vi "SbigExposure.vi"(0 "error in (no error)":errorcluster, 2 "Sbig":T1, 5 "Exposure Time (10ms)":u32, 6 "CCD":u16(ring) items=["CCD IMAGING", "CCD TRACKING"], 7 "Shutter":u16(ring)=1 items=["SHUT LEAVE", "SHUT LIGHT", "SHUT DARK"], 8 "ABG State":u16(ring) items=["ABG OFF", "ABG LOW", "ABG MEDIUM", "ABG HIGH"]) -> (3 "error out":errorcluster)   [LabVIEW 2009]
uses:
  Controls/SbigReference.ctl
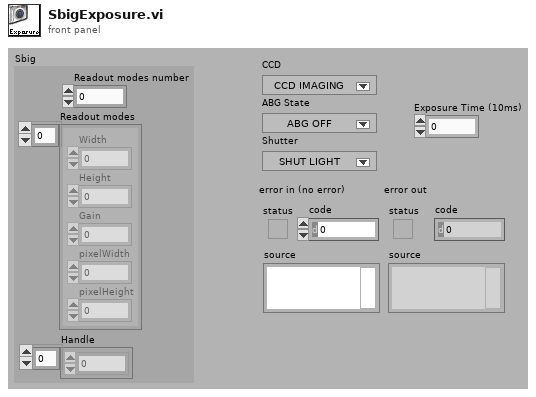
[diagram p1: front panel]
types:
  T1 = typedef "SbigReference.ctl" = cluster{"Readout modes number":u16, "Readout modes":cluster{"Width":u16, "Height":u16, "Gain":dbl, "pixelWidth":dbl, "pixelHeight":dbl}[], "Handle":u16[]}
  T2 = enum16{"0-NoCommand", "1-StartExposure", "2-EndExposure", "3-ReadoutLine", "4-DumpLines", "5-SetTemperatureRegulation", "6-QueryTemperatureStatus", "7-ActivateRelay", "8-PulseOut", "9-EstablishLink", "10-GetDriverInfo", "11-GetCCDInfo", "12-QueryCommandStatus", "13-MiscellaneousControl", "14-ReadSubstractLine", "15-UpdateClock", "16-ReadOffset", "17-OpenDriver", "18-CloseDriver", "19-TXSerialBytes", "20-GetSerialStatus", "21-AOTipTilt", "22-AOSetFocus", "23-AODelay", "24-GetTurboStatus", "25-EndReadout", "26-GetUSTimer", "27-OpenDevice", "28-CloseDevice", "29-SetIRQL", "30-GetIRQL", "31-GetLine", "32-GetLinkStatus", "33-GetDriverHandle", "34-SetDriverHandle", "35-StartReadout", "36-GetErrorString", "37-SetDriverControl", "38-GetDriverControl", "39-USBADControl", "40-QueryUSB", "41-GetPentiumCycleCount", "42-RWUSBI2C", "43-CFW"}
  T3 = enum16{"0-NoCommand", "1-StartExposure", "2-EndExposure", "3-ReadoutLine", "4-DumpLines", "5-SetTemperatureRegulation", "6-QueryTemperatureStatus", "7-ActivateRelay", "8-PulseOut", "9-EstablishLink", "10-GetDriverInfo", "11-GetCCDInfo", "12-QueryCommandStatus", "13-MiscellaneousControl", "14-ReadSubstractLine", "15-UpdateClock", "16-ReadOffset", "17-OpenDriver", "18-CloseDriver", "19-TXSerialBytes", "20-GetSerialStatus", "21-AOTipTilt", "22-AOSetFocus", "23-AODelay", "24-GetTurboStatus", "25-EndReadout", "26-GetUSTimer", "27-OpenDevice", "28-CloseDevice", "29-SetIRQL", "30-GetIRQL", "31-GetLine", "32-GetLinkStatus", "33-GetDriverHandle", "34-SetDriverHandle", "35-StartReadout", "36-GetErrorString", "37-SetDriverControl", "38-GetDriverControl", "39-USBADControl", "40-QueryUSB", "41-GetPentiumCycleCount", "42-RWUSBI2C", "43-CFW"}[]
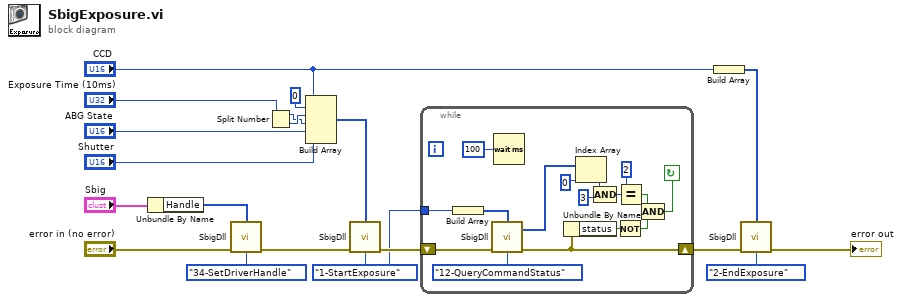
[diagram p0: block diagram]
diagram:
  w6 = T2."1-StartExposure" ("Command")
  n1 = Unbundle By Name("Sbig") -> ("Handle"=w1:u16[])
  n2 = call "SbigDll.vi"("error in (no error)"="error in (no error)", "Command"=T2."34-SetDriverHandle", "Parameters"=w1) -> ("error out"=w3:errorcluster)  [unwired: 1 in, 3 out]
  n3 = Split Number(x="Exposure Time (10ms)") -> (hi(x)=w8:u16, lo(x)=w9:u16)
  n4 = Build Array("CCD", u16 0 ("Elément d'entrée"), w9, w8, "ABG State", "Shutter") -> (w10:u16[])
  n5 = call "SbigDll.vi"("error in (no error)"=w3, "Command"=w6, "Parameters"=w10) -> ("error out"=w14:errorcluster)  [unwired: 1 in, 3 out]
  n6 = while {
    shift-left: w14 -> [w32]
    shift-right: [w23] -> w15
    tunnel: w6 -> [w34]
    stop <- w21 continue-if-true
    n7 = Build Array(w34) -> (w35:T3)
    n8 = call "SbigDll.vi"("error in (no error)"=w32, "Command"=T2."12-QueryCommandStatus", "Parameters"=w35) -> ("error out"=w23:errorcluster, "Results Out"=w26:u16[])  [unwired: 1 in, 2 out]
    n9 = Wait (ms)(milliseconds to wait=u32 100 ("attente (ms)")) -> ()  [unwired: 1 out]
    n10 = Unbundle By Name(w23) -> ("status"=w24:bool)
    n11 = Index Array(array=w26, index=0 ("Indice")) -> (element=w27:u16)
    n12 = Compound Arithmetic op=AND(w27, u16 3 ("Entrée")) -> (w30:u16)
    n13 = Not(x=w24) -> (.not. x?=w22:bool)
    n14 = Equal?(x=u16 2, y=w30) -> (x = y?=w25:bool)
    n15 = Compound Arithmetic op=AND(w25, w22) -> (w21:bool)
  }
  n16 = Build Array("CCD") -> (w17:u16[])
  n17 = call "SbigDll.vi"("error in (no error)"=w15, "Command"=T2."2-EndExposure", "Parameters"=w17) -> ("error out"=→"error out":errorcluster)  [unwired: 1 in, 3 out]
